vi "mathToBotSpeak.vi"(8 "Numeric":dbl, 9 "Params":T1(array[cluster]), 10 "String in":string, 11 "Command":string) -> (2 "resulting string":string)   [LabVIEW 2012]
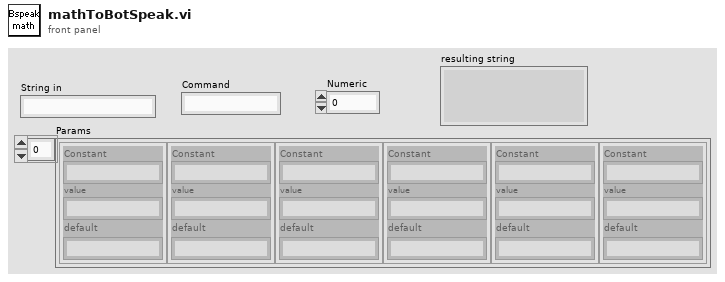
[diagram p1: front panel]
types:
  T1 = cluster{"Constant":string, "value":string, "default":string}[]
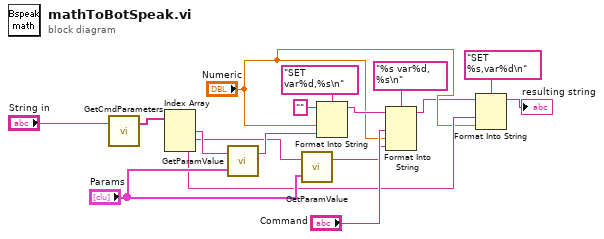
[diagram p0: block diagram]
diagram:
  n1 = call <userlib>:"GetCmdParameters.vi"("Contents"="String in") -> ("variables"=w16:string[])  [unwired: 2 in]
  n2 = Index Array(array=w16) -> (element #1=w12:string, element #2=w10:string, element #3=w5:string)  [unwired: 3 in]
  n3 = call <userlib>:"GetParamValue.vi"("Params"="Params", "command"=w12) -> ("value"=w11:string)  [unwired: 1 out]
  n4 = call <userlib>:"GetParamValue.vi"("Params"="Params", "command"=w10) -> ("value"=w6:string)  [unwired: 1 out]
  n5 = Format Into String(format string="SET var%d,%s\n", initial string="", "Numeric", w11) -> (resulting string=w13:string)  [unwired: 1 in, 1 out]
  n6 = Format Into String(format string="%s var%d, %s\n", initial string=w13, "Command", "Numeric", w6) -> (resulting string=w3:string)  [unwired: 1 in, 1 out]
  n7 = Format Into String(format string="SET %s,var%d\n", initial string=w3, w5, "Numeric") -> (resulting string=→"resulting string":string)  [unwired: 1 in, 1 out]
